vi "to_xml.vi"(8 "error in":errorcluster, 9 "HP83712B Synthesized CW Generator Array":T1, 10 "HP8662A Synthesized Signal Generator Array":T1, 11 "HP83623A Generator Settings Array":T3) -> (0 "error out":errorcluster, 3 "Spectrum Analyzer Settings string":string)   [LabVIEW 2012, in "GPIB.lvclass"]
doc: "Saves analog output settings into xml in the format:\n\n<Enable>%b</Enable>\n<PhysicalChannel>%s</PhysicalChannel>\n<MinimumValue>%f</MinimumValue>\n<MaximumValue>%f</MaximumValue>\n<SamplesPerSecond>%f</SamplesPerSecond>\n<TotalAOTime units=\"seconds\">%s</TotalAOTime>\n<AnalogOutputEquations>\n%s</AnalogOutputEquations>\n<StartTrigger.WaitForStartTrigger>%b</StartTrigger.WaitForStartTrigger\n<StartTrigger.source>%s</StartTrigger.source>\n<StartTrigger.edge>%s</StartTrigger.edge>\n\nMTL 2012 Dec 31"
uses:
  GPIB.lvclass
  HP83623A_RF_Generator/HP83623A_settings.ctl
  RF_Generator_settings_array.ctl
  RF_Generator_settings.ctl
  HP83623A_RF_Generator/HP83623A_RF_Generator.lvclass
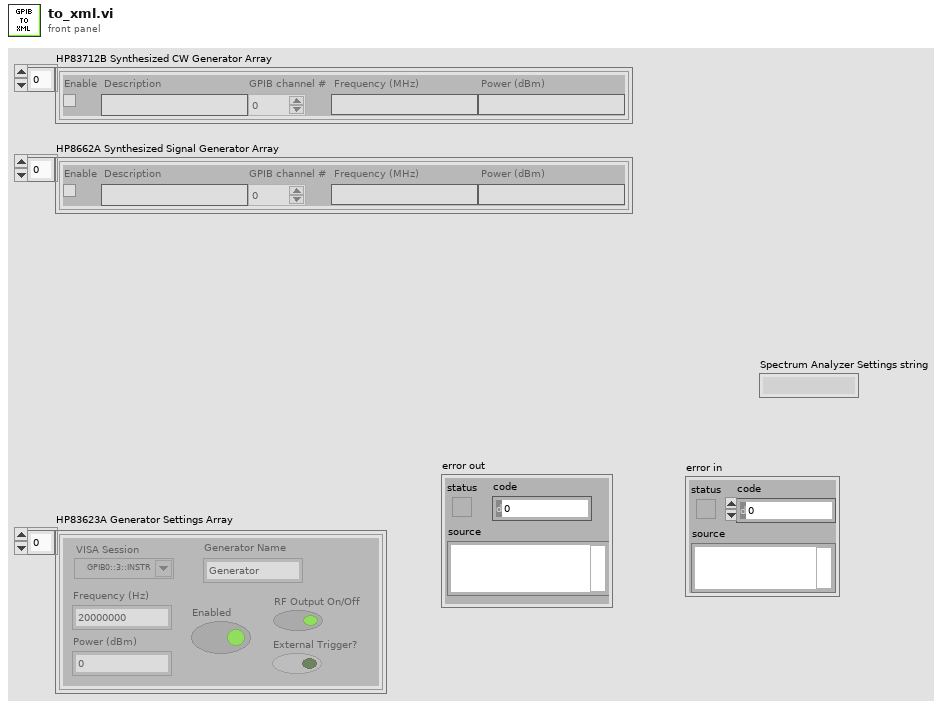
[diagram p1: front panel]
types:
  T1 = typedef "GPIB.lvclass/RF_Generator_settings_array.ctl" = T2[]
  T2 = typedef "GPIB.lvclass/RF_Generator_settings.ctl" = cluster{"Enable":bool, "Description":string, "GPIB channel #":u8, "Frequency (MHz)":string, "Power (dBm)":string}
  T3 = typedef "HP83623A_RF_Generator.lvclass/HP83623A_settings.ctl" = cluster{"Frequency (Hz)":string, "Power (dBm)":string, "Enabled":bool, "initialized":bool, "RF Output On/Off":bool, "External Trigger?":bool, "VISA Session":refnum<visa-resource-name>, "Generator Name":string}[]
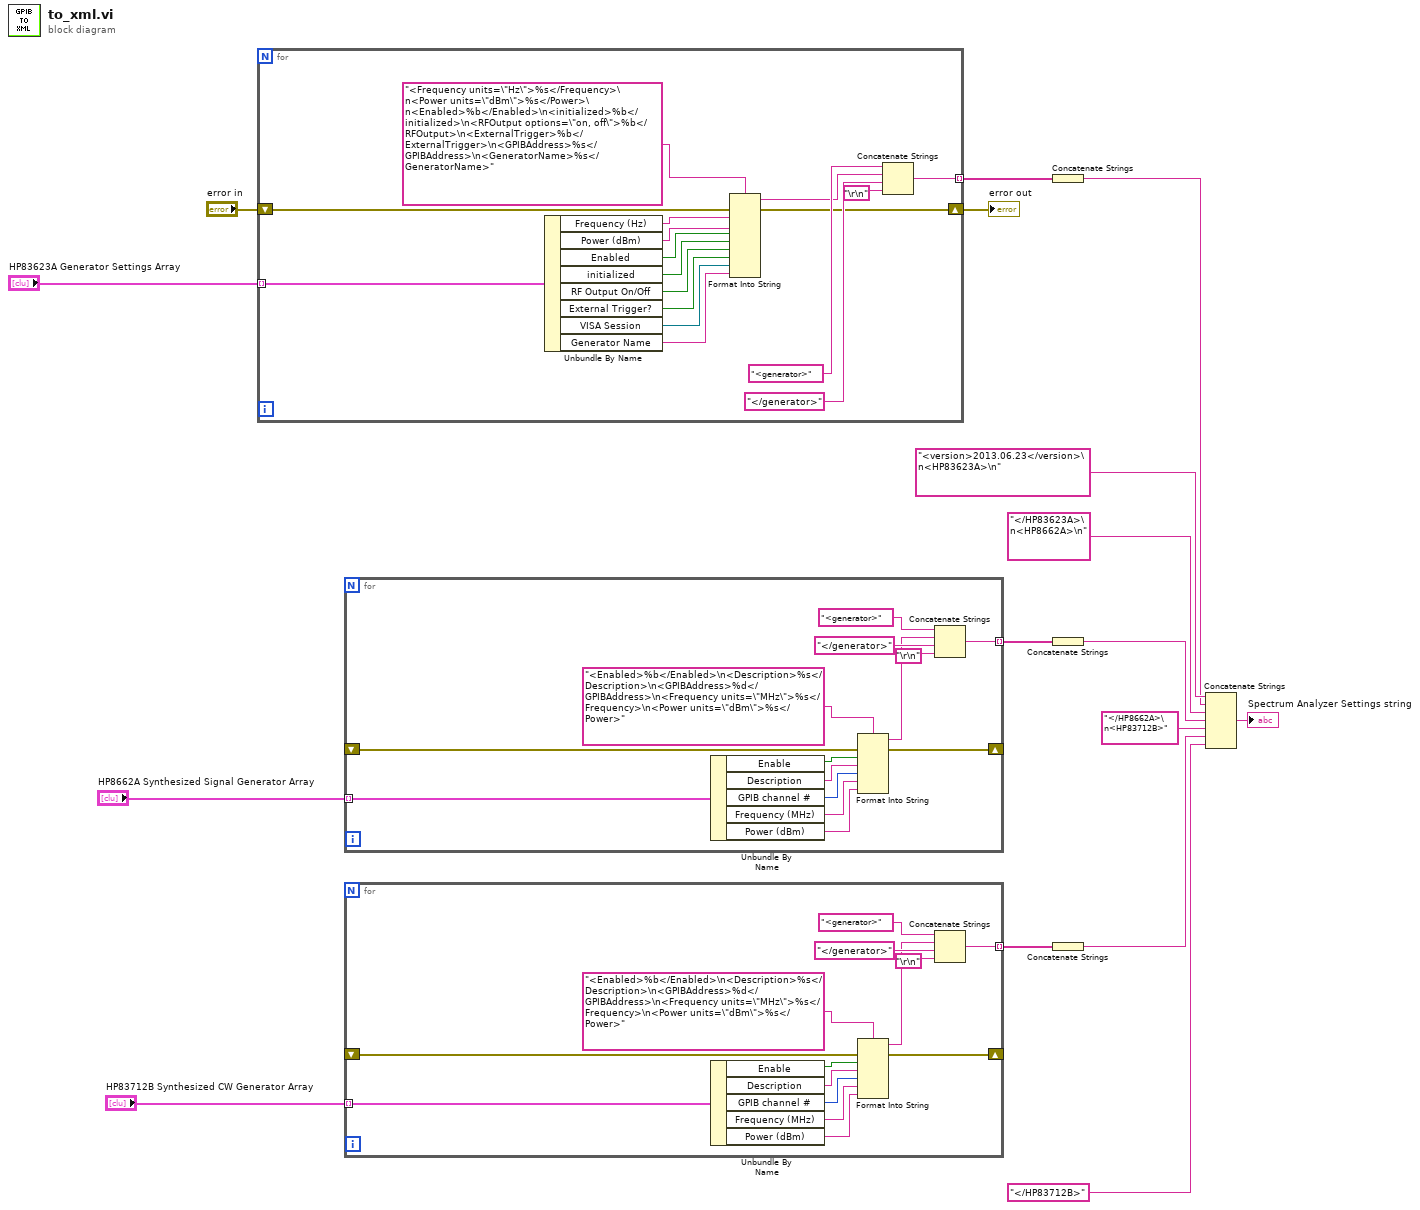
[diagram p0: block diagram]
diagram:
  n1 = for {
    tunnel: "HP83623A Generator Settings Array" -> [w29] mode=indexing
    tunnel: [w33] -> w13 mode=indexing
    shift-right: [w17] -> w14
    shift-left: "error in" -> [w19]
    n2 = Unbundle By Name(w29) -> ("Frequency (Hz)"=w28:string, "Power (dBm)"=w27:string, "Enabled"=w26:bool, "initialized"=w25:bool, "RF Output On/Off"=w24:bool, "External Trigger?"=w23:bool, "VISA Session"=w22:refnum<visa-resource-name>, "Generator Name"=w21:string)
    n3 = Format Into String(format string="<Frequency units=\"Hz\">%s</Frequency>\n<Power units=\"dBm\">%s</Power>\n<Enabled>%b</Enabled>\n<initialized>%b</initialized>\n<RFOutput options=\"on, off\">%b</RFOutput>\n<ExternalTrigger>%b</ExternalTrigger>\n<GPIBAddress>%s</GPIBAddress>\n<GeneratorName>%s</GeneratorName>", error in=w19, w28, w27, w26, w25, w24, w23, w22, w21) -> (resulting string=w18:string, error out=w17:errorcluster)  [unwired: 1 in]
    n4 = Concatenate Strings("<generator>" ("string"), w18, "</generator>" ("string"), "\r\n") -> (w33:string)
  }
  "error out" <- w14
  n5 = for {
    tunnel: "HP8662A Synthesized Signal Generator Array" -> [w43] mode=indexing
    tunnel: [w47] -> w8 mode=indexing
    shift-right: [w34] -> _
    shift-left: _ -> [w36]
    n6 = Unbundle By Name(w43) -> ("Enable"=w42:bool, "Description"=w41:string, "GPIB channel #"=w40:u8, "Frequency (MHz)"=w39:string, "Power (dBm)"=w38:string)
    n7 = Format Into String(format string="<Enabled>%b</Enabled>\n<Description>%s</Description>\n<GPIBAddress>%d</GPIBAddress>\n<Frequency units=\"MHz\">%s</Frequency>\n<Power units=\"dBm\">%s</Power>", error in=w36, w42, w41, w40, w39, w38) -> (resulting string=w35:string, error out=w34:errorcluster)  [unwired: 1 in]
    n8 = Concatenate Strings("<generator>" ("string"), w35, "</generator>" ("string"), "\r\n") -> (w47:string)
  }
  n9 = for {
    tunnel: "HP83712B Synthesized CW Generator Array" -> [w57] mode=indexing
    tunnel: [w61] -> w3 mode=indexing
    shift-right: [w48] -> _
    shift-left: _ -> [w50]
    n10 = Unbundle By Name(w57) -> ("Enable"=w56:bool, "Description"=w55:string, "GPIB channel #"=w54:u8, "Frequency (MHz)"=w53:string, "Power (dBm)"=w52:string)
    n11 = Format Into String(format string="<Enabled>%b</Enabled>\n<Description>%s</Description>\n<GPIBAddress>%d</GPIBAddress>\n<Frequency units=\"MHz\">%s</Frequency>\n<Power units=\"dBm\">%s</Power>", error in=w50, w56, w55, w54, w53, w52) -> (resulting string=w49:string, error out=w48:errorcluster)  [unwired: 1 in]
    n12 = Concatenate Strings("<generator>" ("string"), w49, "</generator>" ("string"), "\r\n") -> (w61:string)
  }
  n13 = Concatenate Strings(w13) -> (w11:string)
  n14 = Concatenate Strings(w8) -> (w7:string)
  n15 = Concatenate Strings(w3) -> (w2:string)
  n16 = Concatenate Strings("<version>2013.06.23</version>\n<HP83623A>\n" ("string"), w11, "</HP83623A>\n<HP8662A>\n" ("string"), w7, "</HP8662A>\n<HP83712B>" ("string"), w2, "</HP83712B>" ("string")) -> (→"Spectrum Analyzer Settings string":string)
